vi "Verify Command Status.vi"(7 "Response Token":string, 11 "Response":string) -> (0 "error out":errorcluster, 3 "Data":string)   [LabVIEW 2012, in "NFC Driver.lvlib"]
uses:
  NFC Driver.lvlib
  <vilib>/Utility/error.llb/Error Cluster From Error Code.vi
  <vilib>/ErrorRing/Error Ring.xnode
panel:
  out "match + rest of string":string
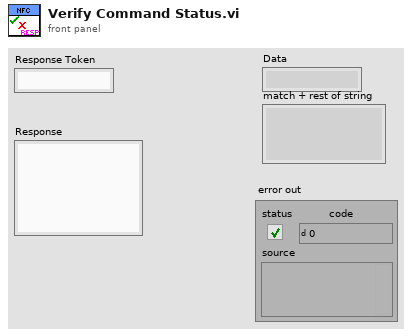
[diagram p1: front panel]
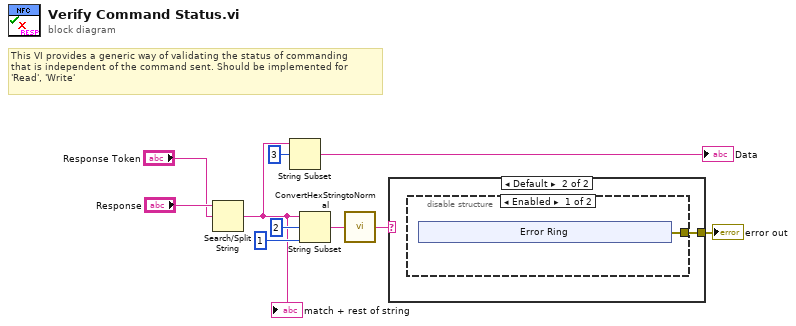
[diagram p0: block diagram]
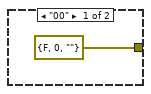
[diagram p2: hidden frame]
diagram:
  # "This VI provides a generic way of validating the status of commanding\nthat is independent of the command sent. Should be implemented for\n'Read', 'Write'"
  n1 = Search/Split String(string="Response", search string/char (-)="Response Token") -> (match + rest of string=w4:string)  [unwired: 1 in, 2 out]
  "match + rest of string" <- w4
  n2 = String Subset(string=w4, offset (0)=3) -> (substring=→"Data":string)  [unwired: 1 in]
  n3 = String Subset(string=w4, offset (0)=2, length (rest)=1 ("length (rest)")) -> (substring=w7:string)
  n4 = call "ConvertHexStringtoNormal.vi"("Hex String"=w7) -> ("Normal String"=w6:string)
  n5 = case shown="Default" w6 {
    tunnel: [errorcluster {"status"=FALSE, "code"=0, "source"=""} ("error out") w12] -> w5
    frame "00" {
    }
    frame Default {
      n6 = disable-structure shown="Enabled" {
        disable-tunnel: [w13 _] -> w12
        frame Enabled {
          n7 = xnode "Error Ring"() -> ("error out"=w13:errorcluster)
        }
        frame Disabled {
          # "we don't check the error bit since it returns error\nintermitently. As long as the rest of the bytes \nare complete, it is valid"
        }
      }
    }
  }
  "error out" <- w5
